vi "getBuffer.vi"(9 "Numeric 3":i32, 10 "Numeric in":dbl, 11 "Array":dbl[](array[numeric])) -> (3 "Numeric out":dbl)   [LabVIEW 2011]
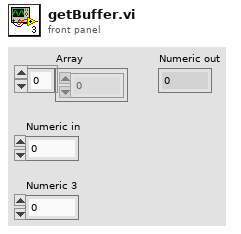
[diagram p1: front panel]
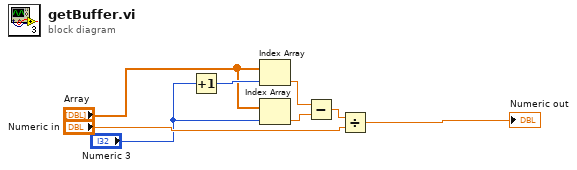
[diagram p0: block diagram]
diagram:
  n1 = Increment(x="Numeric 3") -> (x+1=w3:i32)
  n2 = Index Array(array="Array", index=w3) -> (element=w4:dbl)
  n3 = Index Array(array="Array", index="Numeric 3") -> (element=w5:dbl)
  n4 = Subtract(x=w4, y=w5) -> (x-y=w6:dbl)
  n5 = Divide(x=w6, y="Numeric in") -> (x/y=→"Numeric out":dbl)
